vi "ReceiveVelocityProfile.vi"(5 "VelocityProfile Input":cluster{"position":dbl, "velocity":dbl}, 6 "Timeout ms":i32=1, 7 "UDP Input":T1) -> (0 "Error Out":errorcluster, 1 "VelocityProfile Output":cluster{"position":dbl, "velocity":dbl}, 2 "Did Receive":bool, 3 "UDP Output":T1)   [LabVIEW 2016]
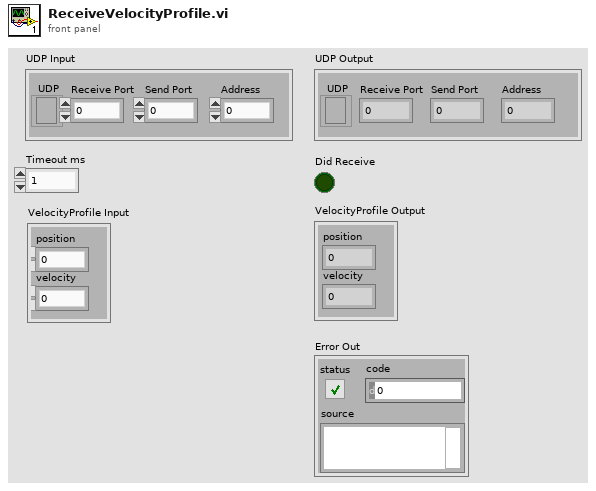
[diagram p1: front panel]
types:
  T1 = cluster{"UDP":refnum<k16>, "Receive Port":i32, "Send Port":i32, "Address":i64}
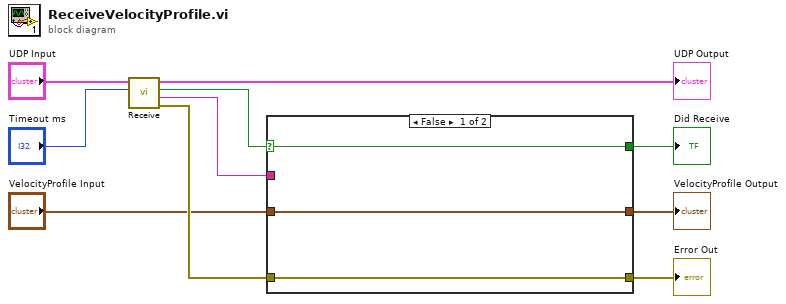
[diagram p0: block diagram]
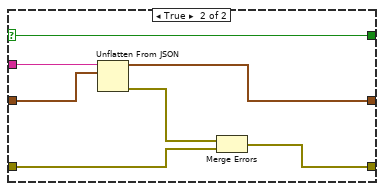
[diagram p2: hidden frame]
diagram:
  n1 = call "Receive.vi"("Timeout ms"="Timeout ms", "UDP Input"="UDP Input") -> ("Error Out"=w7:errorcluster, "Received Data"=w3:string, "Did Receive"=w5:bool, "UDP Output"=→"UDP Output":T1)  [unwired: 2 in]
  n2 = case shown="False" w5 {
    selector: w5 -> [w11 w15]
    tunnel: "VelocityProfile Input" -> [w13 w20]
    tunnel: [w12 w18] -> w6
    tunnel: [w13 w19] -> w1
    tunnel: w7 -> [w12 w16]
    tunnel: [w11 w15] -> w4
    tunnel: w3 -> [_ w14]
    frame False {
    }
    frame True {
      n3 = Unflatten From JSON(JSON string=w14, type and defaults=w20) -> (value=w19:cluster{"position":dbl, "velocity":dbl}, error out=w17:errorcluster)  [unwired: 5 in]
      n4 = Merge Errors(w17, w16) -> (w18:errorcluster)
    }
  }
  "Error Out" <- w6
  "Did Receive" <- w4
  "VelocityProfile Output" <- w1
